vi "labview 96113026.vi"() -> ()   [LabVIEW 2018]
uses:
  <vilib>/Instr/_visa.llb/VISA Configure Serial Port (Instr).vi
panel:
  in  "Tab Control":enum32{"Page 1", "Page 2"}(tab)
  in  "Stop Button":bool
  in  "Start":bool
  out "Response":string
  in  "?":refnum<visa-resource-name>="COM1"
  out "read buffer":string
  out "decimal integer string":string
  in  "baud rate (9600)":u32=9600
  in  "Boolean":bool
  out "Temperature":dbl(slide) scale=0.0..50.0
  out "Humidity":dbl(knob) scale=20.0..100.0
  out "fasele":dbl(knob) scale=0.332..332.0
  out "noor 2":dbl(knob) scale=0.0..1000.0
  out "temp":dbl
  out "humadi":dbl
  in  "relay":bool
  out "value 3":dbl
  out "value 2":dbl
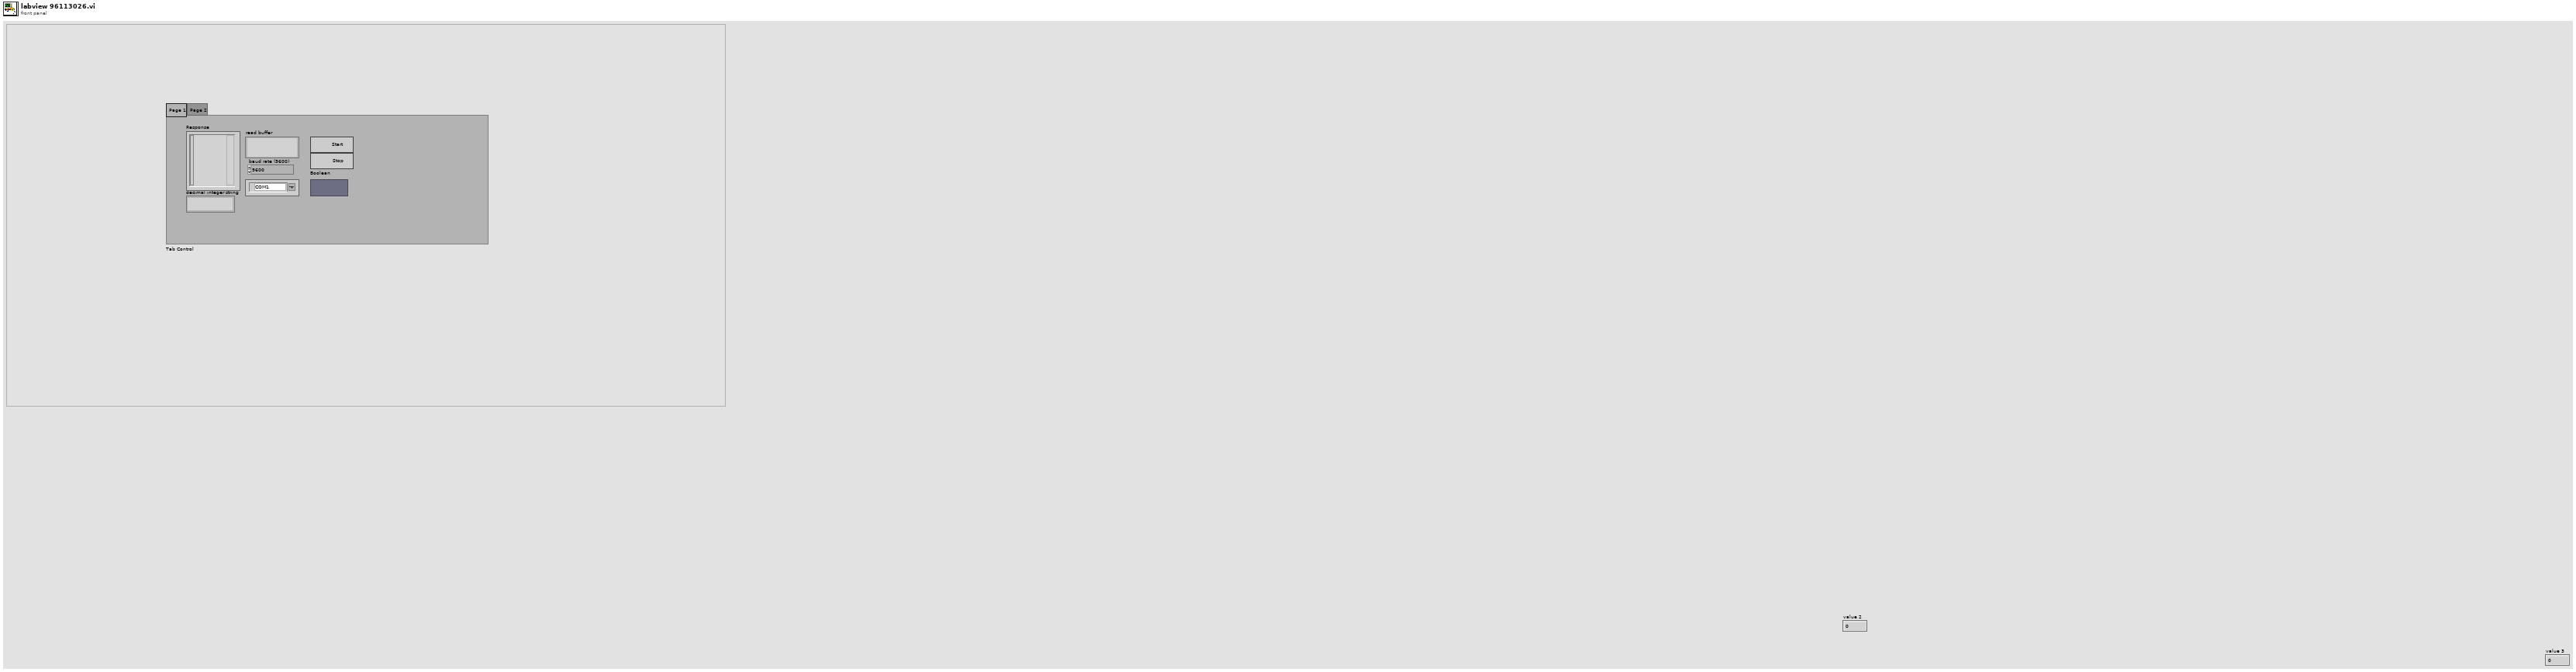
[diagram p1: front panel]
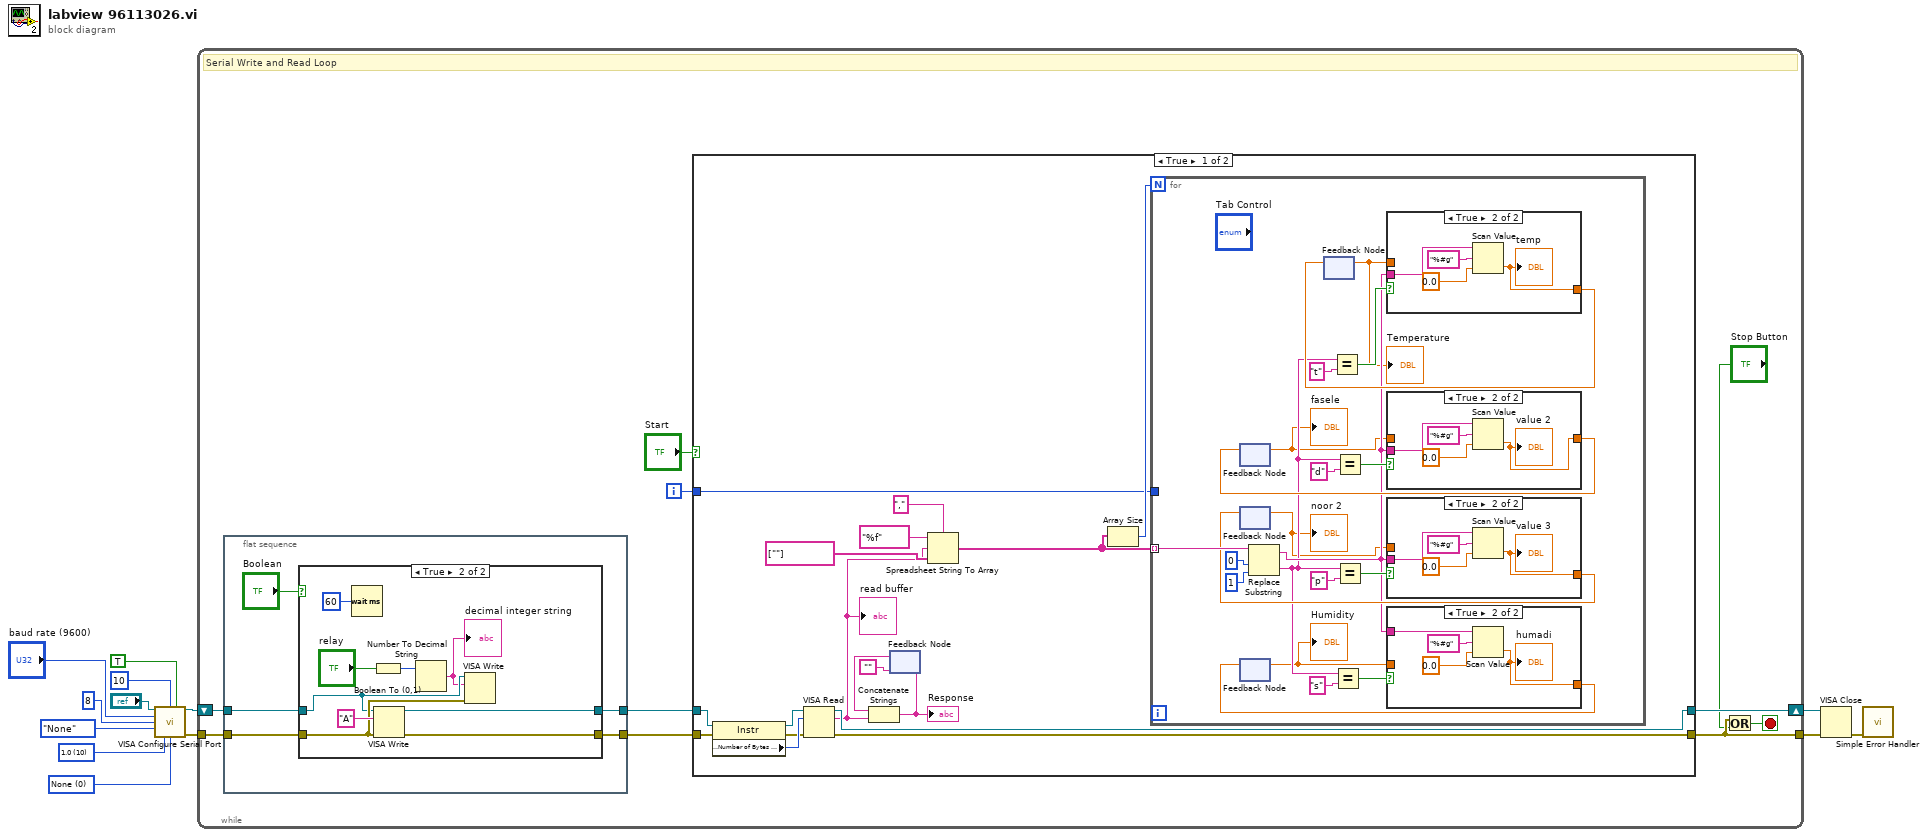
[diagram p0: block diagram]
diagram:
  w6 = u16 0 items=["None", "XON/XOFF", "RTS/CTS", "XON/XOFF & RTS/CTS", "DTR/DSR", "XON/XOFF & DTR/DSR"] ("flow control (0:none)")
  w7 = u16 10 items=["1.0"=10, "1.5"=15, "2.0"=20] ("stop bits (10: 1 bit)")
  n1 = call-poly "VISA Configure Serial Port"("VISA resource name"="?", "termination char\n(0xA = '\\n' = LF)"=u8 10 ("termination char\n(0xA = '\\n' = LF)"), "Enable Termination\nChar (T)"=TRUE ("Enable Termination\nChar (T)"), "baud rate (9600)"="baud rate (9600)", "data bits (8)"=u16 8, "parity (0:none)"=enum16{"None", "Odd", "Even", "Mark", "Space"}."None", "stop bits (10: 1 bit)"=w7, "flow control (0:none)"=w6) -> ("VISA resource name out"=w11:refnum<visa-resource-name>, "error out"=w10:errorcluster)  [unwired: 2 in, 4 out]
  n2 = while {
    shift-right: [w23] -> w12
    shift-left: w11 -> [w17]
    tunnel: w10 -> [w16]
    tunnel: [w21] -> w13
    i -> [w20]
    stop <- w22 stop-if-true
    # "Serial Write and Read Loop"
    n3 = flat-sequence {
      tunnel: [w28] -> w19
      tunnel: [w27] -> w18
      tunnel: w17 -> [w26]
      tunnel: w16 -> [w25]
      frame #0 {
        n4 = case shown="True" "Boolean" {
          tunnel: [w30 w38] -> w28
          tunnel: [w29 w37] -> w27
          tunnel: w26 -> [w30 w33]
          tunnel: w25 -> [w29 w34]
          frame False {
          }
          frame True {
            n5 = Wait (ms)(milliseconds to wait=u32 60) -> ()  [unwired: 1 out]
            n6 = Boolean To (0,1)(Boolean="relay") -> (0, 1=w35:i16)
            n7 = VISA Write(VISA resource name=w33, write buffer="A", error in (no error)=w34) -> (VISA resource name out=w38:refnum<visa-resource-name>, error out=w37:errorcluster)  [unwired: 1 out]
            n8 = Number To Decimal String(number=w35) -> (decimal integer string=w31:string)  [unwired: 1 in]
            "decimal integer string" <- w31
            n9 = VISA Write(VISA resource name=w33, write buffer=w31, error in (no error)=w34) -> ()  [unwired: 3 out]
          }
        }
      }
    }
    n10 = case shown="True" "Start" {
      tunnel: [w56 w99] -> w23
      tunnel: w19 -> [w54 w99]
      tunnel: [w55 w98] -> w21
      tunnel: w18 -> [w53 w98]
      tunnel: w20 -> [w42 _]
      frame True {
        n11 = property class="Instr"(reference=w54, error in=w53) -> (reference out=w51:refnum<visa-resource-name>, error out=w50:errorcluster, "Serial Settings:Number of Bytes at Serial Port"=w52:u32)
        n12 = VISA Read(VISA resource name=w51, byte count=w52, error in (no error)=w50) -> (VISA resource name out=w56:refnum<visa-resource-name>, read buffer=w40:string, error out=w55:errorcluster)  [unwired: 1 out]
        "read buffer" <- w40
        n13 = feedback #1("") -> (w49:string)
        n14 = Concatenate Strings(w49, w40) -> (w41:string)
        "Response" <- w41
        n15 = feedback-in #1(w41) -> ()
        n16 = Spreadsheet String To Array(delimiter (Tab)=",", format string="%f", spreadsheet string=w40, array type (2D Dbl)=string[] [""]) -> (array=w43:string[])
        n17 = Array Size(array=w43) -> (size(s)=w44:i32)
        n18 = for {
          N: w44 -> [_]
          tunnel: w43 -> [w72] mode=indexing
          tunnel: w42 -> [_]
          n19 = feedback #2() -> (w58:dbl)  [unwired: 1 in]
          "fasele" <- w58
          n20 = feedback #3() -> (w57:dbl)  [unwired: 1 in]
          "noor 2" <- w57
          n21 = feedback #4() -> (w59:dbl)  [unwired: 1 in]
          "Humidity" <- w59
          n22 = Replace Substring(2:u8 1, 3:u8 0, 5:w72) -> (0:w61:string, 1:w62:string)  [unwired: 1 in]
          n23 = feedback #5() -> (w60:dbl)  [unwired: 1 in]
          "Temperature" <- w60
          n24 = Equal?(x=w61, y="t") -> (x = y?=w77:bool)
          n25 = Equal?(x=w61, y="s") -> (x = y?=w69:bool)
          n26 = Equal?(x=w61, y="d") -> (x = y?=w66:bool)
          n27 = Equal?(x=w61, y="p") -> (x = y?=w63:bool)
          n28 = case shown="True" w77 {
            tunnel: w62 -> [_ w95]
            tunnel: [w93 w94] -> w73
            tunnel: w60 -> [w93 _]
            frame False {
            }
            frame True {
              n29 = Scan Value(string=w95, format string="%#g", default (0 dbl)=0.0) -> (value=w94:dbl)  [unwired: 1 out]
              "temp" <- w94
            }
          }
          n30 = feedback-in #5(w73) -> ()
          n31 = case shown="True" w66 {
            tunnel: w62 -> [_ w85]
            tunnel: [w83 w84] -> w67
            tunnel: w58 -> [w83 _]
            frame False {
            }
            frame True {
              n32 = Scan Value(string=w85, format string="%#g", default (0 dbl)=0.0) -> (value=w84:dbl)  [unwired: 1 out]
              "value 2" <- w84
            }
          }
          n33 = feedback-in #2(w67) -> ()
          n34 = case shown="True" w63 {
            tunnel: w62 -> [_ w80]
            tunnel: [w78 w79] -> w64
            tunnel: w57 -> [w78 _]
            frame False {
            }
            frame True {
              n35 = Scan Value(string=w80, format string="%#g", default (0 dbl)=0.0) -> (value=w79:dbl)  [unwired: 1 out]
              "value 3" <- w79
            }
          }
          n36 = feedback-in #3(w64) -> ()
          n37 = case shown="True" w69 {
            tunnel: w62 -> [_ w90]
            tunnel: [w88 w89] -> w70
            tunnel: w59 -> [w88 _]
            frame False {
            }
            frame True {
              n38 = Scan Value(string=w90, format string="%#g", default (0 dbl)=0.0) -> (value=w89:dbl)  [unwired: 1 out]
              "humadi" <- w89
            }
          }
          n39 = feedback-in #4(w70) -> ()
        }
      }
      frame False {
      }
    }
    n40 = Or(x=w21, y="Stop Button") -> (x .or. y?=w22:bool)
  }
  n41 = VISA Close(VISA resource name=w12, error in (no error)=w13) -> (error out=w3:errorcluster)
  n42 = call <vilib>:"Simple Error Handler.vi"("error in (no error)"=w3) -> ()  [unwired: 1 in, 8 out]
